vi "CryoServer Cmd Show GUI.vi"(8 "error in (no error)":errorcluster, 10 "Show GUI? (False)":bool, 11 "connection ID":refnum<k5>) -> (0 "error out":errorcluster, 3 "connection ID out":refnum<k5>)   [LabVIEW 2024, in "CryoServer.lvclass"]
uses:
  CryoServer.lvclass
panel:
  out "Command Complete":string
  out "Cmd Ack":string
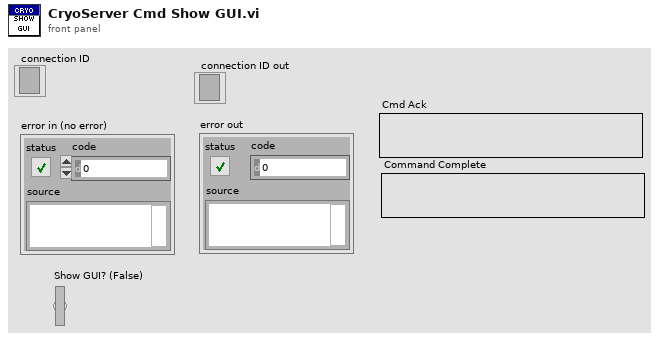
[diagram p1: front panel]
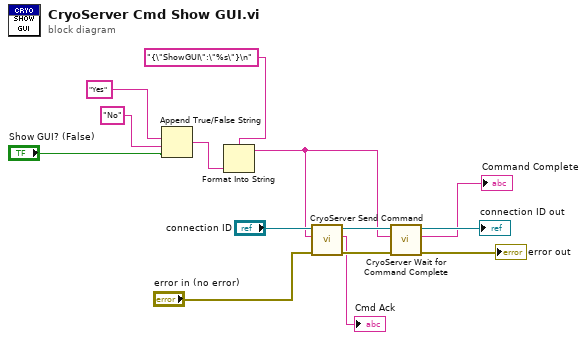
[diagram p0: block diagram]
diagram:
  n1 = Append True/False String(1:"Show GUI? (False)", 2:"No" ("true string"), 3:"Yes" ("true string")) -> (0:w14:string)  [unwired: 1 in]
  n2 = Format Into String(format string="{\"ShowGUI\":\"%s\"}\n", w14) -> (resulting string=w4:string)  [unwired: 2 in, 1 out]
  n3 = call "CryoServer Send Command.vi"("error in (no error)"="error in (no error)", "command string"=w4, "connection ID"="connection ID") -> ("error out"=w7:errorcluster, "Response"=→"Cmd Ack":string, "connection ID out"=w5:refnum<k5>)  [unwired: 6 in]
  n4 = call "CryoServer Wait for Command Complete.vi"("error in (no error)"=w7, "command string"=w4, "connection ID"=w5) -> ("error out"=→"error out":errorcluster, "Response"=→"Command Complete":string, "connection ID out"=→"connection ID out":refnum<k5>)  [unwired: 6 in]
